vi "MPPT Real Time OLD.vi"() -> ()   [LabVIEW 2017]
doc: "This example shows how to create, run a script and query the script output data."
uses:
  <instrlib>/Keithley 2600 Series/Keithley 2600 Series.lvlib
panel:
  in  "stop":bool
  out "XY Graph":cluster{dbl[], dbl[]}(graph)
  out "P(k-1)":dbl
  out "P(k)":dbl
  out "V(k-1)":dbl
  out "V(k)":dbl
  in  "dV":dbl=0.01 caption="limitI"
  in  "Initial Voltage (V)":dbl caption="limitI"
  in  "Current Limit (A)":dbl=0.1 caption="limitI"
  out "TimeStamp":string[](array[string])
  out "Voltage":dbl[](array[numeric])
  out "Current":dbl[](array[numeric])
  out "Power(W)":dbl[](array[numeric])
  in  "USB COM Port":refnum<visa-resource-name>="COM5"
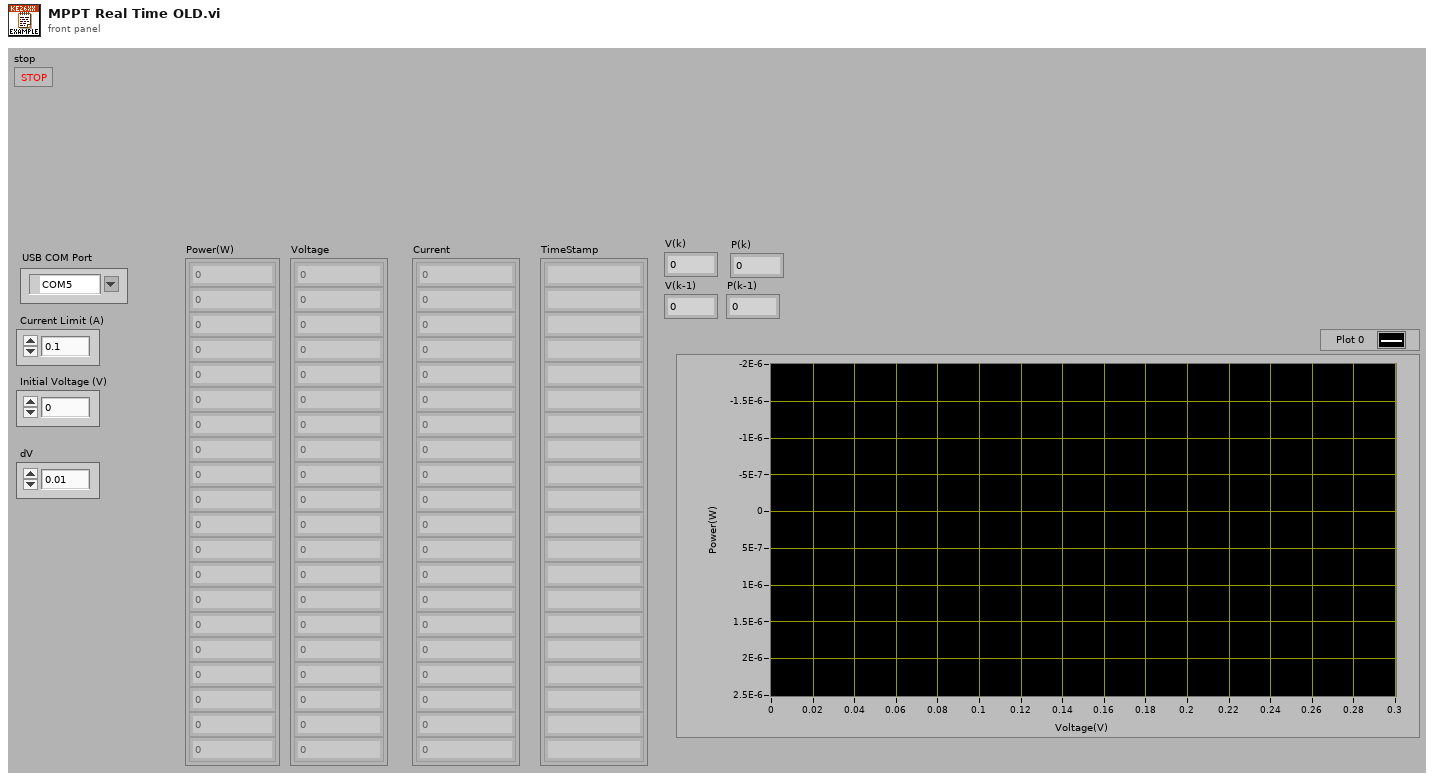
[diagram p1: front panel]
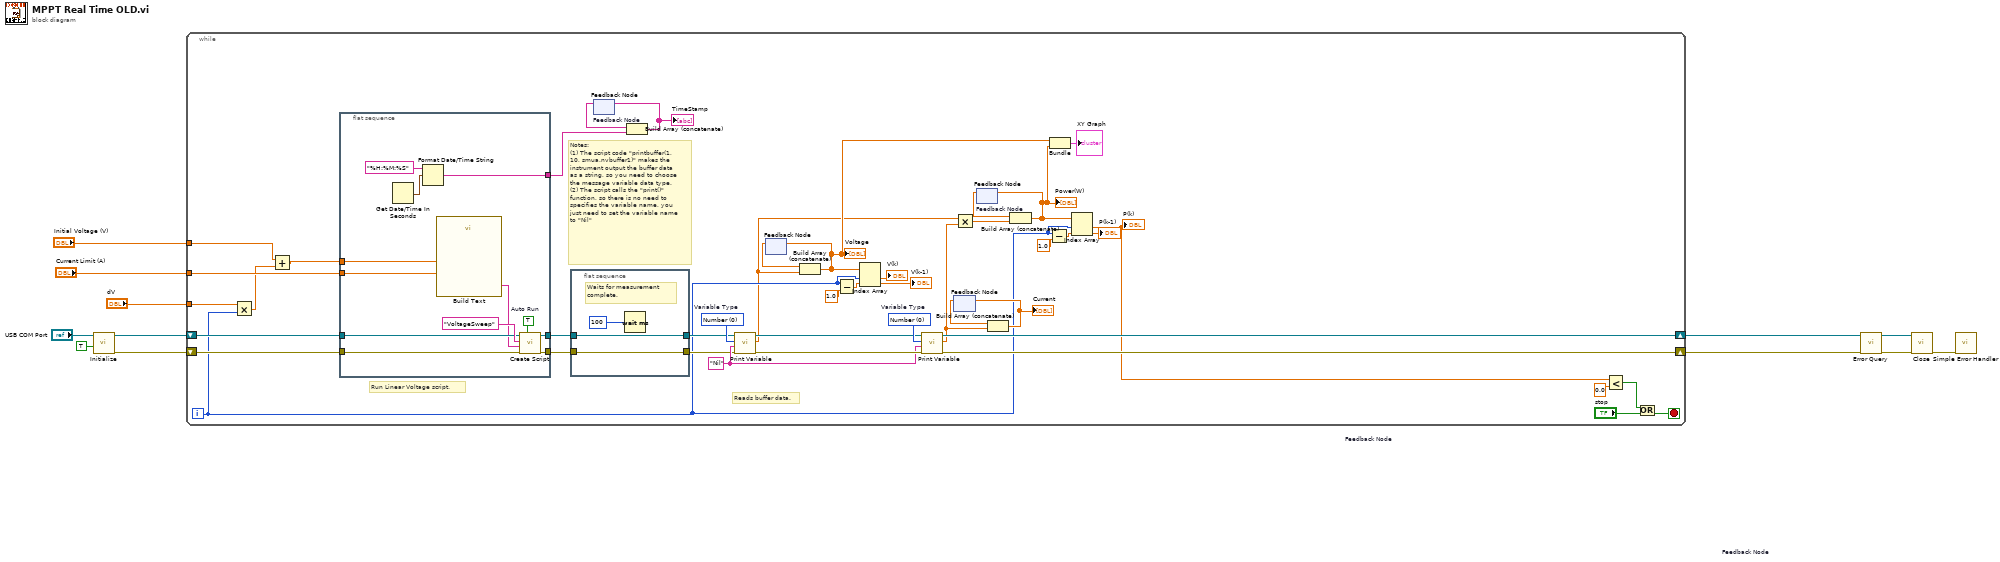
[diagram p0: block diagram]
diagram:
  n1 = call <instrlib>:"Initialize.vi"("Reset (True)"=TRUE, "VISA resource name"="USB COM Port") -> ("error out"=w8:errorcluster, "VISA resource name out"=w9:refnum<visa-resource-name>)  [unwired: 8 in]
  n2 = while {
    tunnel: "Current Limit (A)" -> [w30]
    shift-right: [w48] -> w6
    shift-left: w9 -> [w54]
    shift-right: [w47] -> w5
    shift-left: w8 -> [w53]
    tunnel: "dV" -> [w29]
    tunnel: "Initial Voltage (V)" -> [w27]
    i -> [w19]
    stop <- w17 stop-if-true
    w46 = "Nil"
    w51 = 0 items=["Number", "Message"]  # Variable Type
    w52 = 0 items=["Number", "Message"]  # Variable Type
    # "Reads buffer data."
    # "Notes: \n(1) The script code \"printbuffer(1, 10, smua.nvbuffer1)\" makes the instrument output the buffer data as a string, so you need to choose the message variable data type.\n(2) The script calls the \"print()\" function, so there is no need to specifies the variable name, you just need to set the variable name to \"Nil\""
    # "Run Linear Voltage script."
    n3 = Multiply(x=w29, y=w19) -> (x*y=w28:dbl)
    n4 = Add(x=w27, y=w28) -> (x+y=w26:dbl)
    n5 = flat-sequence {
      tunnel: [w66] -> w56
      tunnel: [w65] -> w55
      tunnel: w54 -> [w64]
      tunnel: w53 -> [w63]
      tunnel: [w59] -> w31
      tunnel: w30 -> [w58]
      tunnel: w26 -> [w57]
      frame #0 {
        w67 = TRUE  # Auto Run
        n6 = Get Date/Time In Seconds() -> (seconds since 1Jan1904=w60:timestamp)
        n7 = Format Date/Time String(time format string (%c)="%H:%M:%S", seconds (now)=w60) -> (date/time string=w59:string)  [unwired: 1 out]
        n8 = call "Build Text"("limitI"=w58, "volt"=w57) -> ("Result"=w62:string)  [unwired: 12 in, 1 out]
        n9 = call <instrlib>:"Create Script.vi"("Auto Run (F: Disable)"=w67, "error in (no error)"=w63, "Source Code"=w62, "Script Variable"="VoltageSweep" ("Script Variable (myScript)"), "VISA resource name"=w64) -> ("error out"=w65:errorcluster, "VISA resource name out"=w66:refnum<visa-resource-name>)  [unwired: 5 in]
      }
    }
    n10 = flat-sequence {
      tunnel: w56 -> [w69]
      tunnel: w55 -> [w70]
      tunnel: [w70] -> w44
      tunnel: [w69] -> w45
      frame #0 {
        # "Waits for measurement complete."
        n11 = Wait (ms)(milliseconds to wait=100 ("Temp Delay")) -> ()  [unwired: 1 out]
      }
    }
    n12 = feedback #1 "Feedback Node"() -> (w32:string[])  [unwired: 1 in]
    n13 = Build Array (concatenate)(w32, w31) -> (w33:string[])
    "TimeStamp" <- w33
    n14 = feedback-in #1(w33) -> ()
    n15 = call <instrlib>:"Print Variable.vi"("error in (no error)"=w44, "Variable Name"=w46, "Variable Type (0: Number)"=w52, "VISA resource name"=w45) -> ("error out"=w49:errorcluster, "Number"=w18:dbl, "VISA resource name out"=w50:refnum<visa-resource-name>)  [unwired: 4 in, 1 out]
    n16 = feedback #2 "Feedback Node"() -> (w41:dbl[])  [unwired: 1 in]
    n17 = Build Array (concatenate)(w41, w18) -> (w24:dbl[])
    "Voltage" <- w24
    n18 = feedback-in #2(w24) -> ()
    n19 = Subtract(x=w19, y=1.0) -> (x-y=w35:dbl)
    n20 = Index Array(array=w24, index #1=w19, index #2=w35) -> (element #1=→"V(k)":dbl, element #2=→"V(k-1)":dbl)
    n21 = call <instrlib>:"Print Variable.vi"("error in (no error)"=w49, "Variable Name"=w46, "Variable Type (0: Number)"=w51, "VISA resource name"=w50) -> ("error out"=w47:errorcluster, "Number"=w38:dbl, "VISA resource name out"=w48:refnum<visa-resource-name>)  [unwired: 4 in, 1 out]
    n22 = feedback #3 "Feedback Node"() -> (w40:dbl[])  [unwired: 1 in]
    n23 = Multiply(x=w18, y=w38) -> (x*y=w42:dbl)
    n24 = feedback #4 "Feedback Node"() -> (w43:dbl[])  [unwired: 1 in]
    n25 = Build Array (concatenate)(w40, w38) -> (w39:dbl[])
    "Current" <- w39
    n26 = feedback-in #3(w39) -> ()
    n27 = Build Array (concatenate)(w43, w42) -> (w25:dbl[])
    "Power(W)" <- w25
    n28 = feedback-in #4(w25) -> ()
    n29 = Subtract(x=w19, y=1.0) -> (x-y=w37:dbl)
    n30 = Bundle(w24, w25) -> (→"XY Graph":cluster{dbl[], dbl[]})  [unwired: 1 in]
    n31 = Index Array(array=w25, index #1=w19, index #2=w37) -> (element #1=w13:dbl, element #2=→"P(k-1)":dbl)
    "P(k)" <- w13
    n32 = Less?(x=w13, y=0.0) -> (x < y?=w15:bool)
    n33 = Or(x=w15, y="stop") -> (x .or. y?=w17:bool)
  }
  n34 = call <instrlib>:"Error Query.vi"("error in (no error)"=w5, "VISA resource name"=w6) -> ("error out"=w11:errorcluster, "VISA resource name out"=w12:refnum<visa-resource-name>)  [unwired: 6 in, 2 out]
  n35 = call <instrlib>:"Close.vi"("error in (no error)"=w11, "VISA resource name"=w12) -> ("error out"=w1:errorcluster)  [unwired: 9 in]
  n36 = call <vilib>:"Simple Error Handler.vi"("error in (no error)"=w1) -> ()  [unwired: 4 in, 5 out]
